vi "UIRef.vi"(8 "error in":errorcluster, 11 "node in":refnum<class "Job Initialize.lvclass">) -> (0 "error out":errorcluster, 2 "VI refnum":refnum<vi>, 3 "node out":refnum<class "Job Initialize.lvclass">)   [LabVIEW 2014, in "Job Initialize.lvclass"]
doc: "Stores the static reference to the UI of the node."
uses:
  Job Initialize.lvclass
  Job Initialize UI.vi
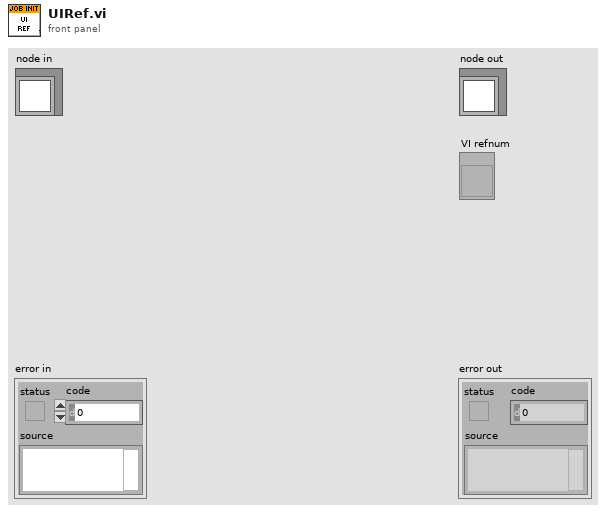
[diagram p1: front panel]
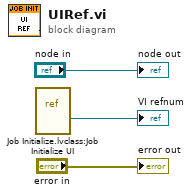
[diagram p0: block diagram]
diagram:
  n1 = vi-ref "Job Initialize.lvclass:Job Initialize UI.vi"() -> (→"VI refnum":refnum<vi>)
  "error out" <- "error in"
  "node out" <- "node in"
